vi "6.3.vi"() -> ()   [LabVIEW 2017]
uses:
  <vilib>/Utility/file.llb/Write Delimited Spreadsheet (DBL).vi
  <vilib>/measure/NI_MABase.lvlib
panel:
  out "Y":dbl[](array[numeric])
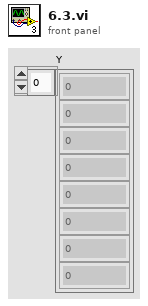
[diagram p1: front panel]
types:
  T1 = enum16{"open", "replace", "create", "open or create", "replace or create", "replace or create with confirmation"}
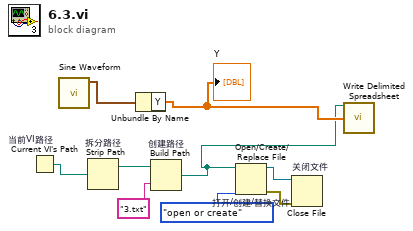
[diagram p0: block diagram]
diagram:
  n1 = Current VI's Path "当前VI路径"() -> (path=w8:path)
  n2 = call <vilib>:"Sine Waveform.vi"() -> ("signal out"=w9:waveform(dbl))  [unwired: 10 in, 1 out]
  n3 = Strip Path "拆分路径"(path=w8) -> (stripped path=w7:path)  [unwired: 1 out]
  n4 = Unbundle By Name(w9) -> ("Y"=w4:dbl[])
  "Y" <- w4
  n5 = Build Path "创建路径"(base path=w7, name or relative path="3.txt") -> (appended path=w3:path)
  n6 = Open/Create/Replace File "打开/创建/替换文件"(file path (use dialog)=w3, operation (0:open)=T1."open or create" ("操作(0:open)")) -> (refnum out=w2:refnum<file>, error out=w1:errorcluster)  [unwired: 4 in, 1 out]
  n7 = Close File "关闭文件"(refnum=w2, error in=w1) -> ()  [unwired: 2 out]
  n8 = call-poly <vilib>:"Write Delimited Spreadsheet.vi"("file path (dialog if empty)"=w3, "1D data"=w4) -> ()  [unwired: 12 in, 2 out]
